vi "Teleop.vi"(10 "Match Info":T2={"Autonomous Elapsed Seconds"=0.0, "TeleOp Elapsed Seconds"=0.0, "Disabled Elapsed Seconds"=0.0, "Visited Autonomous"=FALSE, "Visited TeleOp"=FALSE, "Visited Disabled"=FALSE, "Autonomous Settings"={"Autonomous Style"=enum."Independent", "VI Refnum"=refnum}}, 11 "Call Context":T3) -> ()   [LabVIEW 2012]
doc: "This VI is called for each TeleOp packet received from the DS where the robot is not disabled. It is often used to read from the joysticks and update I/O or to update setpoints for timed control loops. It should complete and return within 20 milliseconds or it may miss DS packets."
uses:
  <vilib>/Rock Robotics/WPI/DriverStation/WPI_DriverStationDerivedRobotMode.ctl
  <vilib>/Rock Robotics/WPI/DriverStation/WPI_DriverStationMatch Info.ctl
  <vilib>/Rock Robotics/WPI/Relay/WPI_RelayValue.ctl
  <vilib>/Rock Robotics/WPI/Solenoid/WPI_SolenoidValue.ctl
  Robot Global Data.vi
  <vilib>/addons/control/pid/pid.llb/PID (DBL).vi
  <vilib>/Rock Robotics/WPI/RobotDrive/WPI_RobotDriveGetSetRefNum.vi
  <vilib>/Rock Robotics/WPI/Joystick/WPI_JoystickGetSetRefNum.vi
  <vilib>/Rock Robotics/WPI/Solenoid/WPI_SolenoidSetEnum.vi
  <vilib>/addons/control/pid/NI_PID_pid.lvlib
panel:
  in  "y 2":dbl=0.59
  in  "y":dbl=0.6
  in  "Boolean":bool
  in  "Time to twitch":dbl=1300.0
  in  "Time of start twitch":dbl
  in  "Turn speed for twitch":dbl=0.7
  in  "Twitch":string="Nope"
  in  "PID Gains Angle":T1={"proportional gain (Kc)"=1.0, "integral time (Ti, min)"=0.01, "derivative time (Td, min)"=0.0} {"derivative time (Td, min)" format="%.3f"; "integral time (Ti, min)" format="%.3f"; "proportional gain (Kc)" format="%.3f"}
  in  "PID Gains for distance":T1={"proportional gain (Kc)"=1.0, "integral time (Ti, min)"=0.01, "derivative time (Td, min)"=0.0} {"derivative time (Td, min)" format="%.3f"; "integral time (Ti, min)" format="%.3f"; "proportional gain (Kc)" format="%.3f"}
  in  "Threshold for shooter":dbl=0.015
  in  "Posistioned":string="Nothing"
  in  "Angle Target":dbl
  out "Distance From Target":dbl
  out "Ready To Fire":bool
  in  "S Off Time":dbl=0.5
  in  "S On Time":dbl=0.2
  in  "Time Last Fired":dbl
  in  "Current Status":string="Roaming"
  in  "Shooter Speed":dbl format="%.2f"
  in  "Shooter On":bool=TRUE
  out "Waveform Chart":cluster{"Rate":dbl, "Rate":dbl}(graph)
  out "Rate 1":dbl
  out "Rate 2":dbl
  in  "PID gains":T1={"proportional gain (Kc)"=1.0, "integral time (Ti, min)"=0.007, "derivative time (Td, min)"=0.0} {"derivative time (Td, min)" format="%.3f"; "integral time (Ti, min)" format="%.3f"; "proportional gain (Kc)" format="%.3f"}
  in  "Maximum Encoder speed":dbl=25000.0
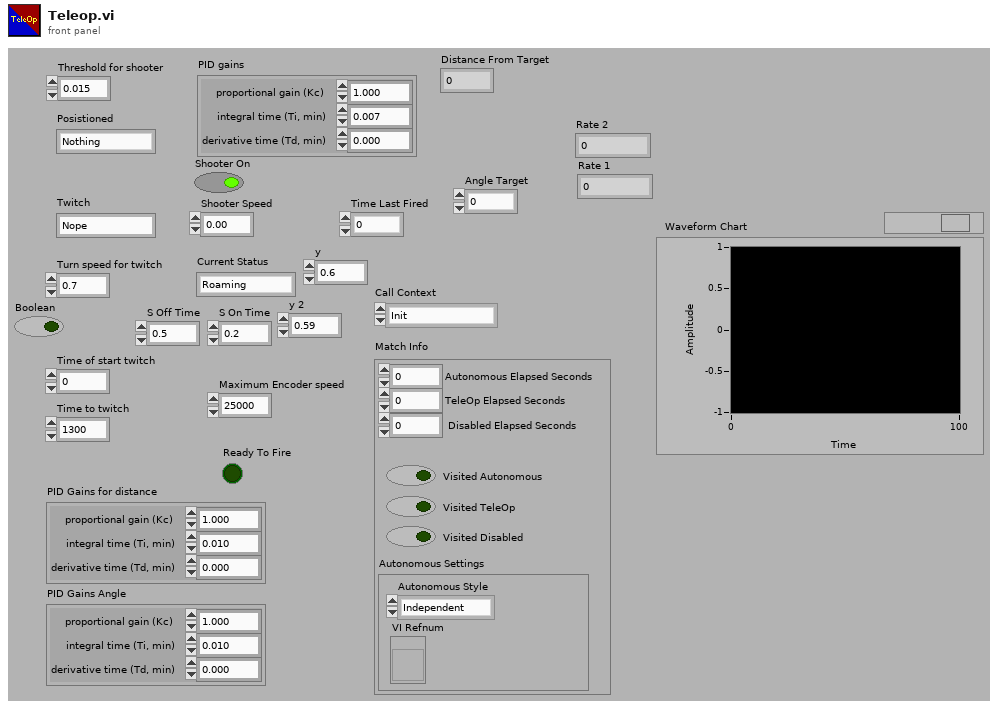
[diagram p1: front panel]
types:
  T1 = cluster{"proportional gain (Kc)":dbl, "integral time (Ti, min)":dbl, "derivative time (Td, min)":dbl}
  T2 = typedef "WPI_DriverStationMatch Info.ctl" = cluster{"Autonomous Elapsed Seconds":dbl, "TeleOp Elapsed Seconds":dbl, "Disabled Elapsed Seconds":dbl, "Visited Autonomous":bool, "Visited TeleOp":bool, "Visited Disabled":bool, "Autonomous Settings":cluster{"Autonomous Style":enum16{"Iterative", "Independent"}, "VI Refnum":refnum<vi>}}
  T3 = typedef "WPI_DriverStationDerivedRobotMode.ctl" = enum16{"Init", "Execute", "Stop"}
  T4 = typedef "WPI_EncoderDevRef.ctl" = cluster{"DevStatus":errorcluster, "EncoderIndex":T5, "CounterIndex":T6, "DistancePerCount":dbl, "Decoding Type":T7}
  T5 = typedef "FPGA_EncoderIdx.ctl" = enum8{"Enc 0", "Enc 1", "Enc 2", "Enc 3", "Invalid"}
  T6 = typedef "FPGA_CounterCtrSystemIndex.ctl" = enum8{"Ctr 0", "Ctr 1", "Ctr 2", "Ctr 3", "Ctr 4", "Ctr 5", "Ctr 6", "Ctr 7", "Invalid"}
  T7 = typedef "WPI_EncoderType.ctl" = enum16{"1x", "2x", "4x"}
  T8 = typedef "WPI_JoystickDevRef.ctl" = cluster{"Device":T9}
  T9 = typedef "WPI_JoystickDeviceEnum.ctl" = enum16{"USB 1", "USB 2", "USB 3", "USB 4", "Kinect 1", "Kinect 2"}
  T10 = typedef "WPI_JoystickButtonState.ctl" = cluster{"Button 1":bool, "Button 2":bool, "Button 3":bool, "Button 4":bool, "Button 5":bool, "Button 6":bool, "Button 7":bool, "Button 8":bool, "Button 9":bool, "Button 10":bool, "Button 11":bool, "Button 12":bool}
  T11 = typedef "WPI_RobotDriveDevRef.ctl" = cluster{"DevStatus":errorcluster, "Motors[]":T12[], "Square Inputs":bool, "Max Output":dbl, "Isochronous":bool}
  T12 = typedef "WPI_MotorControlDeviceRef.ctl" = cluster{"DeviceStatus":errorcluster, "Type":enum16{"PWM", "CAN"}, "PWM":cluster{"Digital Module":T13, "PWM Channel":T14, "DeadBand":T15}, "CAN":cluster{"Device Number":u8, "Control Mode":T16, "Semaphore":T17, "Max Vout":dbl}, "Invert":bool, "TransformRef":T18, "InvTransformRef":T18}
  T13 = typedef "FPGA_TypedefDigitalModule.ctl" = enum16{"Digital Module 1", "Digital Module 2"}
  T14 = typedef "FPGA_DIOPWMChannel.ctl" = enum8{"PWM 1", "PWM 2", "PWM 3", "PWM 4", "PWM 5", "PWM 6", "PWM 7", "PWM 8", "PWM 9", "PWM 10", "Invalid"}
  T15 = typedef "WPI_PWMDeadband.ctl" = cluster{"Name":string, "maxPositivePwm":i32, "minPositivePwm":i32, "centerPwm":i32, "maxNegativePwm":i32, "minNegativePwm":i32, "angularRange":u16}
  T16 = typedef "WPI_CANJaguar_ControlMode.ctl" = enum8{"Percent VBus", "Current", "Speed", "Position", "Voltage"}
  T17 = typedef "Semaphore RefNum" = refnum<k1>
  T18 = typedef "WPI_PWMTransform_ConPane.ctl" = refnum<vi>
  T19 = cluster{"axis 1 (x)":dbl, "axis 2 (y)":dbl, "axis 3 (throttle)":dbl, "axis 4":dbl, "axis 5":dbl, "axis 6":dbl}
  T20 = typedef "WPI_RelayValue.ctl" = enum16{"Off", "On", "Forward", "Reverse"}
  T21 = typedef "WPI_RelayDevRef.ctl" = cluster{"DevStatus":errorcluster, "Relay Channel":T22, "Digital Module":T13, "Relay Direction":T23}
  T22 = typedef "FPGA_DIORelayChannel.ctl" = enum8{"Relay 1", "Relay 2", "Relay 3", "Relay 4", "Relay 5", "Relay 6", "Relay 7", "Relay 8", "Invalid"}
  T23 = typedef "WPI_RelayDirection.ctl" = enum16{"Both directions", "Forward only", "Reverse only"}
  T24 = typedef "WPI_SolenoidValue.ctl" = enum16{"Off", "On", "Forward", "Reverse"}
  T25 = typedef "WPI_SolenoidDevRef.ctl" = cluster{"DevStatus":errorcluster, "Solenoid Module":T26, "Forward Solenoid Channel":T27, "Reverse Solenoid Channel":T27}
  T26 = typedef "FPGA_TypedefSolenoidModule.ctl" = enum16{"Solenoid Module 1", "Solenoid Module 2"}
  T27 = typedef "WPI_SolenoidChannel.ctl" = enum8{"Solenoid 1", "Solenoid 2", "Solenoid 3", "Solenoid 4", "Solenoid 5", "Solenoid 6", "Solenoid 7", "Solenoid 8", "Invalid"}
  T28 = cluster{"Center Position":cluster{"X":dbl, "Y":dbl}, "Distance (ft)":dbl, "Center":bool}[]
  T29 = cluster{"Center Position":cluster{"X":dbl, "Y":dbl}, "Distance (ft)":dbl, "Center":bool}
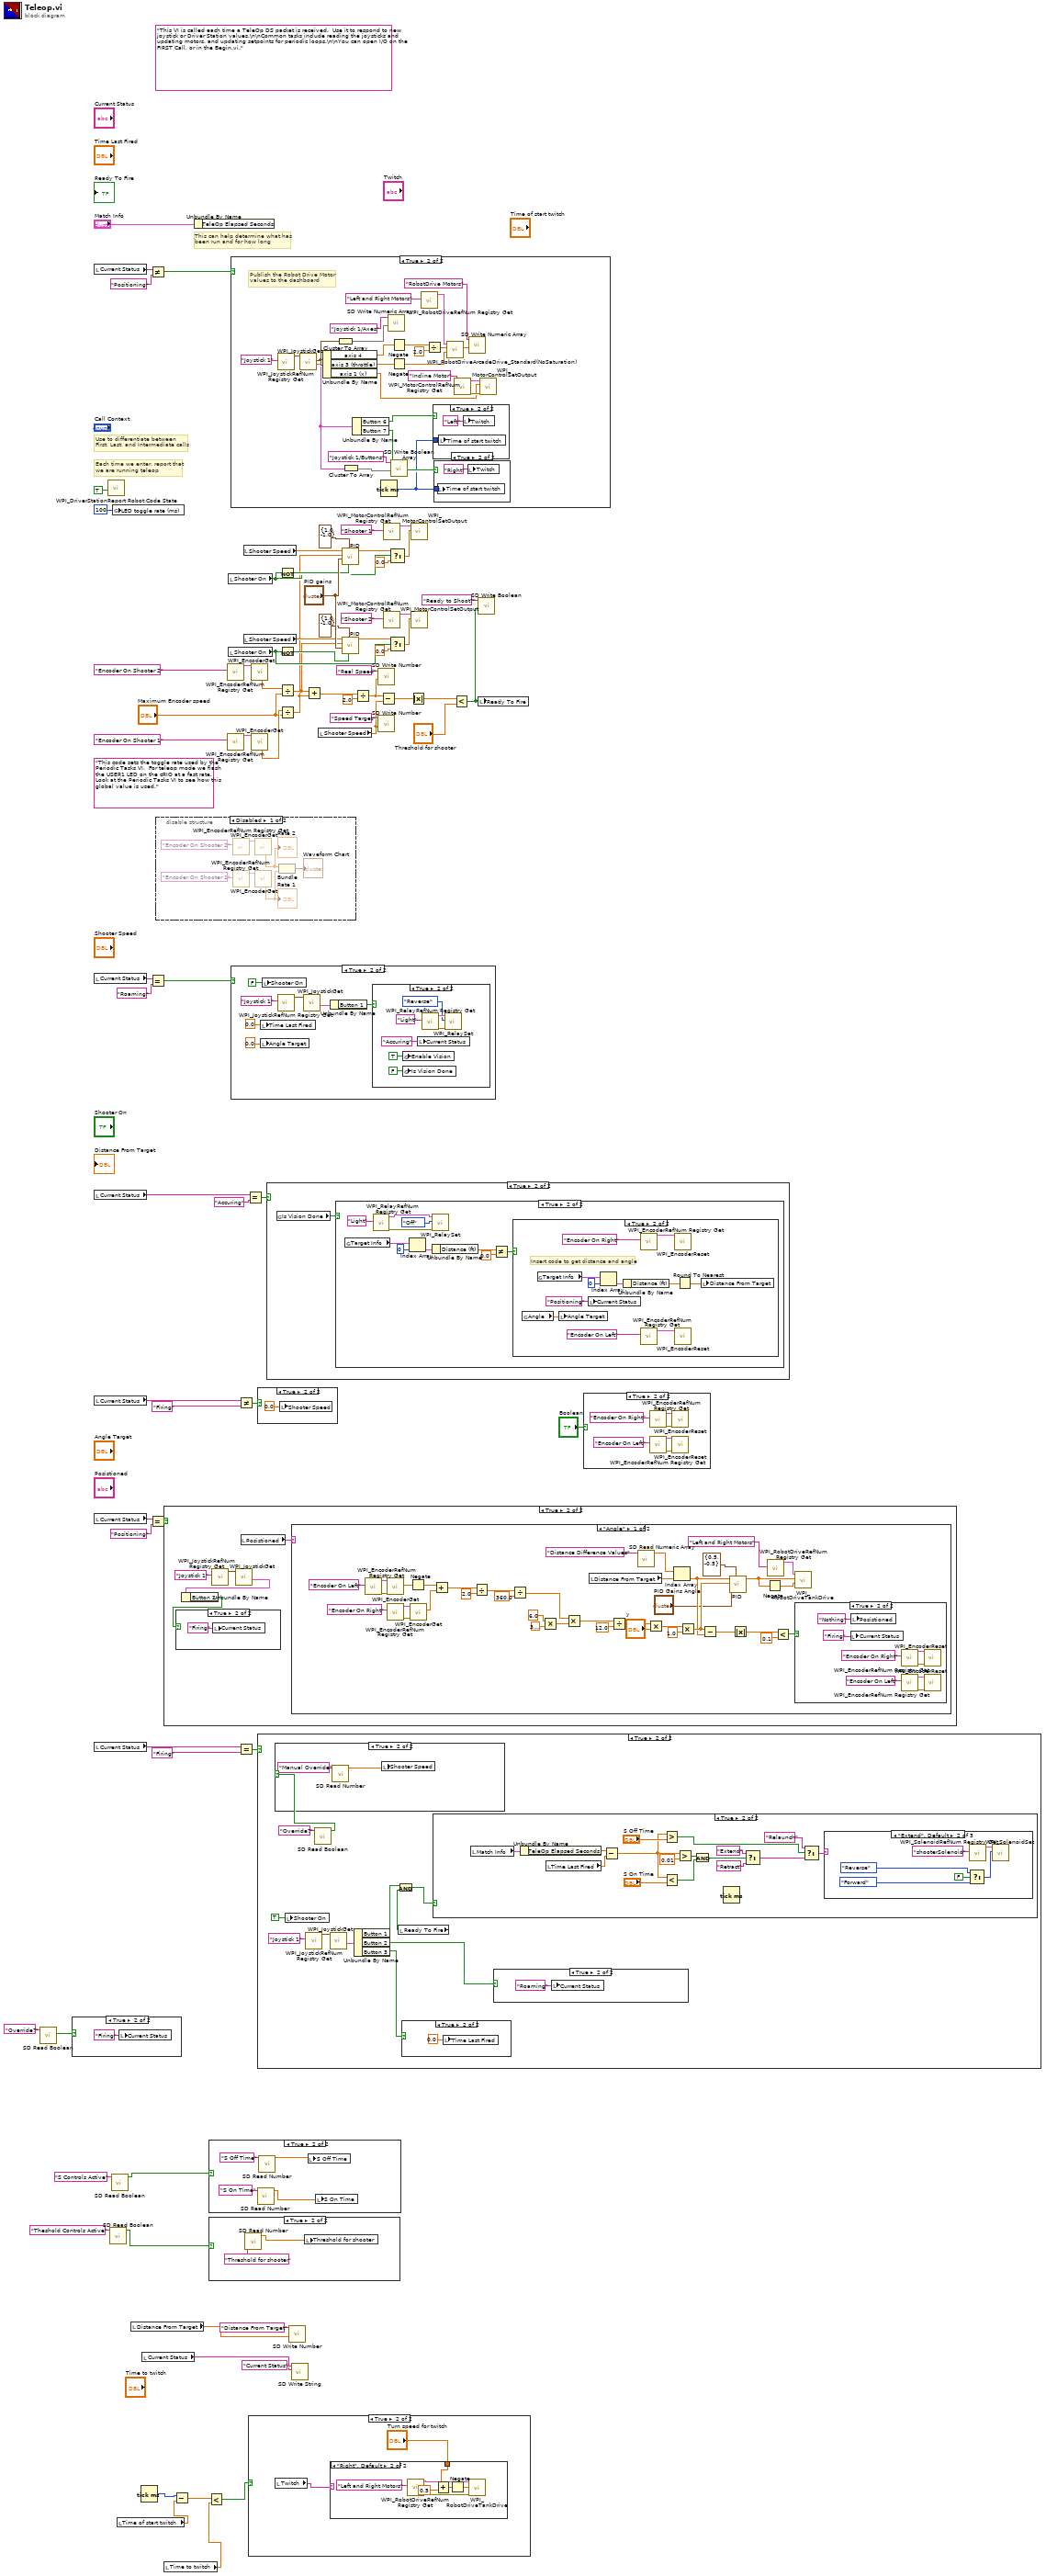
[diagram p0: block diagram]
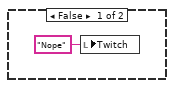
[diagram p3: hidden frame]
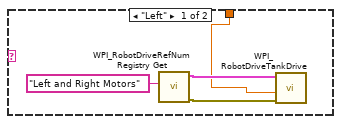
[diagram p4: hidden frame]
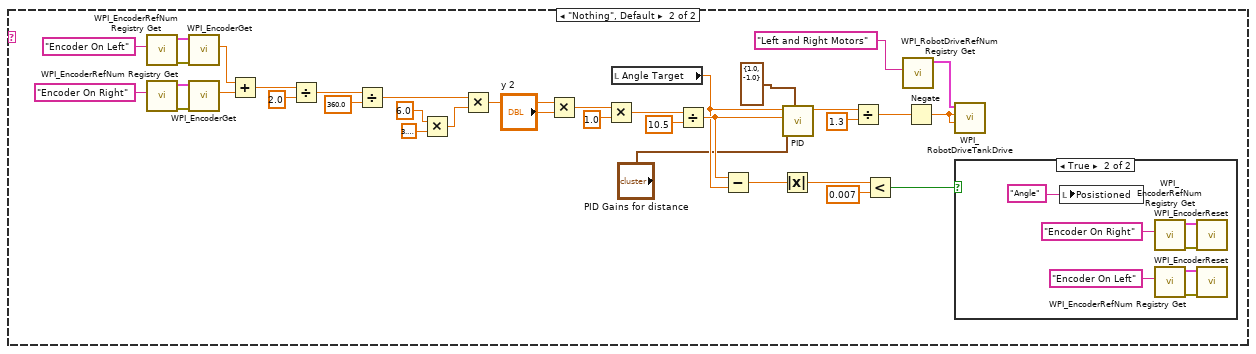
[diagram p12: hidden frame]
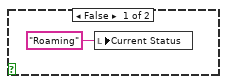
[diagram p19: hidden frame]
diagram:
  (unwired) "This code sets the toggle rate used by the Periodic Tasks VI.  For teleop mode we flash the USER1 LED on the cRIO at a fast rate.  Look at the Periodic Tasks VI to see how this global value is used."
  (unwired) "This VI is called each time a TeleOp DS packet is received.  Use it to respond to new joystick or Driver Station values.\n\nCommon tasks include reading the joysticks and updating motors, and updating setpoints for periodic loops.\n\nYou can open I/O on the FIRST Call, or in the Begin.vi."
  # "Each time we enter, report that\nwe are running teleop"
  # "Use to differentiate between\nFirst, Last, and Intermediate calls"
  # "This can help determine what has\nbeen run and for how long"
  n1 = call <vilib>:"SD Read Boolean.vi"("Name"="Override?") -> ("Boolean"=w15:bool)  [unwired: 8 in, 2 out]
  n2 = case shown="True" w15 {
    frame False {
    }
    frame True {
      n3 = local write "Current Status"("Firing" ("Current Status")) -> ()
    }
  }
  n4 = local read "Current Status"() -> (w26:string)
  n5 = local read "Current Status"() -> (w32:string)
  n6 = local read "Current Status"() -> (w29:string)
  n7 = local read "Current Status"() -> (w19:string)
  n8 = local read "Current Status"() -> (w23:string)
  n9 = local read "Current Status"() -> (w47:string)
  n10 = call <vilib>:"WPI_DriverStationReport Robot Code State.vi"("TeleOp"=TRUE ("Autonomous")) -> ()  [unwired: 10 in, 1 out]
  n11 = call <vilib>:"SD Read Boolean.vi"("Name"="Theshold Controls Active") -> ("Boolean"=w14:bool)  [unwired: 8 in, 2 out]
  n12 = call <vilib>:"SD Read Boolean.vi"("Name"="S Controls Active") -> ("Boolean"=w12:bool)  [unwired: 8 in, 2 out]
  n13 = global write "Robot Global Data.vi" "LED toggle rate (ms)"(u32 100 ("LED ms toggle rate")) -> ()
  n14 = local read "Time of start twitch"() -> (w5:dbl)
  n15 = local read "Distance From Target"() -> (w9:dbl)
  n16 = Tick Count (ms)() -> (millisecond timer value=w6:u32)
  n17 = local read "Current Status"() -> (w7:string)
  n18 = Not Equal?(x=w26, y="Positioning") -> (x != y?=w24:bool)
  n19 = Equal?(x=w32, y="Roaming") -> (x = y?=w30:bool)
  n20 = Equal?(x=w23, y="Positioning") -> (x = y?=w21:bool)
  n21 = disable-structure shown="Disabled" {
    frame Disabled {
      n22 = call <vilib>:"WPI_EncoderRefNum Registry Get.vi"("refnum name"="Encoder On Shooter 2") -> ("EncoderDevRef"=w83:T4)  [unwired: 9 in, 1 out]
      n23 = call <vilib>:"WPI_EncoderRefNum Registry Get.vi"("refnum name"="Encoder On Shooter 1") -> ("EncoderDevRef"=w82:T4)  [unwired: 9 in, 1 out]
      n24 = call <vilib>:"WPI_EncoderGet.vi"("EncoderDevRef"=w83) -> ("Rate"=w80:dbl)  [unwired: 5 in, 5 out]
      "Rate 2" <- w80
      n25 = call <vilib>:"WPI_EncoderGet.vi"("EncoderDevRef"=w82) -> ("Rate"=w81:dbl)  [unwired: 5 in, 5 out]
      "Rate 1" <- w81
      n26 = Bundle("Rate"=w80, "Rate"=w81) -> (→"Waveform Chart":cluster{"Rate":dbl, "Rate":dbl})  [unwired: 1 in]
    }
    frame Enabled {
    }
  }
  n27 = case shown="True" w21 {
    frame False {
    }
    frame True {
      n28 = call <vilib>:"WPI_JoystickRefNum Registry Get.vi"("refnum name"="Joystick 1") -> ("JoystickDevRef"=w87:T8)  [unwired: 9 in, 1 out]
      n29 = call <vilib>:"WPI_JoystickGet.vi"("JoystickDevRef"=w87) -> ("Buttons"=w86:T10)  [unwired: 4 in, 2 out]
      n30 = Unbundle By Name(w86) -> ("Button 2"=w85:bool)
      n31 = case shown="True" w85 {
        frame False {
        }
        frame True {
          n32 = local write "Current Status"("Firing" ("Current Status")) -> ()
        }
      }
      n33 = local read "Posistioned"() -> (w89:string)
      n34 = case shown="\"Angle\"" w89 {
        frame "Angle" {
          n35 = call <vilib>:"WPI_EncoderRefNum Registry Get.vi"("refnum name"="Encoder On Left") -> ("error out"=w104:errorcluster, "EncoderDevRef"=w105:T4)  [unwired: 9 in]
          n36 = call <vilib>:"WPI_EncoderGet.vi"("error in (no error)"=w104, "EncoderDevRef"=w105) -> ("Distance"=w97:dbl)  [unwired: 4 in, 5 out]
          n37 = call <vilib>:"WPI_EncoderRefNum Registry Get.vi"("refnum name"="Encoder On Right") -> ("error out"=w106:errorcluster, "EncoderDevRef"=w107:T4)  [unwired: 9 in]
          n38 = Negate(x=w97) -> (-x=w96:dbl)
          n39 = call <vilib>:"WPI_EncoderGet.vi"("error in (no error)"=w106, "EncoderDevRef"=w107) -> ("Distance"=w110:dbl)  [unwired: 4 in, 5 out]
          n40 = Add(x=w96, y=w110) -> (x+y=w111:dbl)
          n41 = Divide(x=w111, y=2.0) -> (x/y=w115:dbl)
          n42 = Divide(x=w115, y=360.0) -> (x/y=w117:dbl)
          n43 = Multiply(x=6.0, y=3.141592653589793) -> (x*y=w118:dbl)
          n44 = Multiply(x=w117, y=w118) -> (x*y=w119:dbl)
          n45 = local read "Distance From Target"() -> (w94:dbl)
          n46 = Divide(x=w119, y=12.0) -> (x/y=w100:dbl)
          n47 = call <vilib>:"SD Read Numeric Array.vi"("Name"="Distance Difference Values") -> ("Numeric Array"=w124:dbl[])  [unwired: 8 in, 2 out]
          n48 = Multiply(x=w100, y="y") -> (x*y=w99:dbl)
          n49 = Index Array(array=w124, index=w94) -> (element=w93:dbl)
          n50 = Multiply(x=w99, y=1.0) -> (x*y=w95:dbl)
          n51 = Subtract(x=w95, y=w93) -> (x-y=w125:dbl)
          n52 = call-poly <vilib>:"PID.vi"("output range"=cluster{"output high":dbl, "output low":dbl} {"output high"=0.5, "output low"=-0.5}, "PID gains"="PID Gains Angle", "process variable"=w95, "setpoint"=w93) -> ("output"=w101:dbl)  [unwired: 6 in, 1 out]
          n53 = Absolute Value(x=w125) -> (abs(x)=w126:dbl)
          n54 = Negate(x=w101) -> (-x=w103:dbl)
          n55 = call <vilib>:"WPI_RobotDriveRefNum Registry Get.vi"("refnum name"="Left and Right Motors") -> ("RobotDriveDevRef"=w122:T11)  [unwired: 9 in, 1 out]
          n56 = Less?(x=w126, y=0.1) -> (x < y?=w128:bool)
          n57 = call <vilib>:"WPI_RobotDriveTankDrive.vi"("Right axis value"=w103, "Left axis value"=w101, "RobotDriveDevRef"=w122) -> ()  [unwired: 6 in, 3 out]
          n58 = case shown="True" w128 {
            frame False {
            }
            frame True {
              n59 = local write "Current Status"("Firing" ("Current Status")) -> ()
              n60 = local write "Posistioned"("Nothing" ("Posistioned")) -> ()
              n61 = call <vilib>:"WPI_EncoderRefNum Registry Get.vi"("refnum name"="Encoder On Right") -> ("error out"=w134:errorcluster, "EncoderDevRef"=w135:T4)  [unwired: 9 in]
              n62 = call <vilib>:"WPI_EncoderRefNum Registry Get.vi"("refnum name"="Encoder On Left") -> ("error out"=w132:errorcluster, "EncoderDevRef"=w133:T4)  [unwired: 9 in]
              n63 = call <vilib>:"WPI_EncoderReset.vi"("error in (no error)"=w134, "EncoderDevRef"=w135) -> ()  [unwired: 8 in, 2 out]
              n64 = call <vilib>:"WPI_EncoderReset.vi"("error in (no error)"=w132, "EncoderDevRef"=w133) -> ()  [unwired: 8 in, 2 out]
            }
          }
        }
        frame "Nothing", Default {
          n65 = call <vilib>:"WPI_EncoderRefNum Registry Get.vi"("refnum name"="Encoder On Left") -> ("error out"=w172:errorcluster, "EncoderDevRef"=w171:T4)  [unwired: 9 in]
          n66 = call <vilib>:"WPI_EncoderRefNum Registry Get.vi"("refnum name"="Encoder On Right") -> ("error out"=w170:errorcluster, "EncoderDevRef"=w169:T4)  [unwired: 9 in]
          n67 = call <vilib>:"WPI_EncoderGet.vi"("error in (no error)"=w172, "EncoderDevRef"=w171) -> ("Distance"=w166:dbl)  [unwired: 4 in, 5 out]
          n68 = call <vilib>:"WPI_EncoderGet.vi"("error in (no error)"=w170, "EncoderDevRef"=w169) -> ("Distance"=w148:dbl)  [unwired: 4 in, 5 out]
          n69 = Add(x=w166, y=w148) -> (x+y=w165:dbl)
          n70 = Divide(x=w165, y=2.0) -> (x/y=w161:dbl)
          n71 = Divide(x=w161, y=360.0) -> (x/y=w154:dbl)
          n72 = Multiply(x=6.0, y=3.141592653589793) -> (x*y=w159:dbl)
          n73 = Multiply(x=w154, y=w159) -> (x*y=w143:dbl)
          n74 = Multiply(x=w143, y="y 2") -> (x*y=w142:dbl)
          n75 = Multiply(x=w142, y=1.0) -> (x*y=w141:dbl)
          n76 = local read "Angle Target"() -> (w139:dbl)
          n77 = Divide(x=w141, y=10.5) -> (x/y=w150:dbl)
          n78 = Subtract(x=w150, y=w139) -> (x-y=w151:dbl)
          n79 = Absolute Value(x=w151) -> (abs(x)=w152:dbl)
          n80 = call-poly <vilib>:"PID.vi"("output range"=cluster{"output high":dbl, "output low":dbl} {"output high"=1.0, "output low"=-1.0}, "PID gains"="PID Gains for distance", "process variable"=w150, "setpoint"=w139) -> ("output"=w155:dbl)  [unwired: 6 in, 1 out]
          n81 = Divide(x=w155, y=1.3) -> (x/y=w147:dbl)
          n82 = Less?(x=w152, y=0.007) -> (x < y?=w145:bool)
          n83 = call <vilib>:"WPI_RobotDriveRefNum Registry Get.vi"("refnum name"="Left and Right Motors") -> ("RobotDriveDevRef"=w156:T11)  [unwired: 9 in, 1 out]
          n84 = Negate(x=w147) -> (-x=w146:dbl)
          n85 = call <vilib>:"WPI_RobotDriveTankDrive.vi"("Right axis value"=w146, "Left axis value"=w146, "RobotDriveDevRef"=w156) -> ()  [unwired: 6 in, 3 out]
          n86 = case shown="True" w145 {
            frame False {
            }
            frame True {
              n87 = local write "Posistioned"("Angle" ("Posistioned")) -> ()
              n88 = call <vilib>:"WPI_EncoderRefNum Registry Get.vi"("refnum name"="Encoder On Right") -> ("error out"=w175:errorcluster, "EncoderDevRef"=w174:T4)  [unwired: 9 in]
              n89 = call <vilib>:"WPI_EncoderRefNum Registry Get.vi"("refnum name"="Encoder On Left") -> ("error out"=w177:errorcluster, "EncoderDevRef"=w176:T4)  [unwired: 9 in]
              n90 = call <vilib>:"WPI_EncoderReset.vi"("error in (no error)"=w175, "EncoderDevRef"=w174) -> ()  [unwired: 8 in, 2 out]
              n91 = call <vilib>:"WPI_EncoderReset.vi"("error in (no error)"=w177, "EncoderDevRef"=w176) -> ()  [unwired: 8 in, 2 out]
            }
          }
        }
      }
    }
  }
  n92 = local read "Time to twitch"() -> (w3:dbl)
  n93 = Subtract(x=w6, y=w5) -> (x-y=w4:dbl)
  n94 = Unbundle By Name("Match Info") -> ()  [unwired: 1 out]
  n95 = Less?(x=w4, y=w3) -> (x < y?=w2:bool)
  n96 = case shown="True" w12 {
    frame False {
    }
    frame True {
      n97 = call <vilib>:"SD Read Number.vi"("Name"="S On Time") -> ("Numeric"=w182:dbl)  [unwired: 8 in, 2 out]
      n98 = call <vilib>:"SD Read Number.vi"("Name"="S Off Time") -> ("Numeric"=w183:dbl)  [unwired: 8 in, 2 out]
      n99 = local write "S Off Time"(w183) -> ()
      n100 = local write "S On Time"(w182) -> ()
    }
  }
  n101 = case shown="True" w14 {
    frame False {
    }
    frame True {
      n102 = call <vilib>:"SD Read Number.vi"("Name"="Threshold for shooter") -> ("Numeric"=w184:dbl)  [unwired: 8 in, 2 out]
      n103 = local write "Threshold for shooter"(w184) -> ()
    }
  }
  n104 = call <vilib>:"WPI_EncoderRefNum Registry Get.vi"("refnum name"="Encoder On Shooter 2") -> ("EncoderDevRef"=w61:T4)  [unwired: 9 in, 1 out]
  n105 = call <vilib>:"WPI_EncoderRefNum Registry Get.vi"("refnum name"="Encoder On Shooter 1") -> ("EncoderDevRef"=w70:T4)  [unwired: 9 in, 1 out]
  n106 = local read "Shooter On"() -> (w50:bool)
  n107 = local read "Shooter On"() -> (w51:bool)
  n108 = case shown="True" w24 {
    frame False {
    }
    frame True {
      # "Publish the Robot Drive Motor\nvalues to the dashboard"
      n109 = call <vilib>:"WPI_JoystickRefNum Registry Get.vi"("refnum name"="Joystick 1") -> ("JoystickDevRef"=w203:T8)  [unwired: 1 in, 9 out]
      n110 = call <vilib>:"WPI_JoystickGet.vi"("JoystickDevRef"=w203) -> ("Buttons"=w189:T10, "Axes"=w206:T19)  [unwired: 1 in, 4 out]
      n111 = Unbundle By Name(w206) -> ("axis 4"=w199:dbl, "axis 3 (throttle)"=w197:dbl, "axis 1 (x)"=w190:dbl)
      n112 = Cluster To Array(cluster=w206) -> (array=w207:dbl[])
      n113 = Cluster To Array(cluster=w189) -> (array=w204:bool[])
      n114 = Unbundle By Name(w189) -> ("Button 6"=w188:bool, "Button 7"=w187:bool)
      n115 = Tick Count (ms)() -> (millisecond timer value=w186:u32)
      n116 = call <vilib>:"SD Write Numeric Array.vi"("Numeric Array"=w207, "Name"="Joystick 1/Axes") -> ()  [unwired: 8 in, 2 out]
      n117 = Negate(x=w199) -> (-x=w196:dbl)
      n118 = Negate(x=w197) -> (-x=w198:dbl)
      n119 = call <vilib>:"SD Write Boolean Array.vi"("Boolean Array"=w204, "Name"="Joystick 1/Buttons") -> ()  [unwired: 8 in, 2 out]
      n120 = call <vilib>:"WPI_RobotDriveRefNum Registry Get.vi"("refnum name"="Left and Right Motors") -> ("RobotDriveDevRef"=w202:T11)  [unwired: 1 in, 9 out]
      n121 = Divide(x=w196, y=2.0) -> (x/y=w194:dbl)
      n122 = case shown="True" w188 {
        tunnel: w186 -> [_ w211]
        frame False {
        }
        frame True {
          n123 = local write "Time of start twitch"(w211) -> ()
          n124 = local write "Twitch"("Left" ("Twitch")) -> ()
        }
      }
      n125 = case shown="True" w187 {
        tunnel: w186 -> [_ w213]
        frame False {
        }
        frame True {
          n126 = local write "Time of start twitch"(w213) -> ()
          n127 = local write "Twitch"("Right" ("Twitch")) -> ()
        }
      }
      n128 = call <vilib>:"WPI_RobotDriveArcadeDrive_Standard(NoSaturation).vi"("Y axis value"=w198, "X axis value"=w194, "RobotDriveDevRef"=w202) -> ("Motor Values"=w210:dbl[])  [unwired: 1 in, 7 out]
      n129 = call <vilib>:"WPI_MotorControlRefNum Registry Get.vi"("refnum name"="Incline Motor") -> ("error out"=w192:errorcluster, "MotorControlDevRef"=w191:T12)  [unwired: 9 in]
      n130 = call <vilib>:"SD Write Numeric Array.vi"("Numeric Array"=w210, "Name"="RobotDrive Motors") -> ()  [unwired: 8 in, 2 out]
      n131 = call <vilib>:"WPI_MotorControlSetOutput.vi"("error in (no error)"=w192, "Output"=w190, "MotorControlDevRef"=w191) -> ()  [unwired: 6 in, 3 out]
    }
  }
  n132 = case shown="True" w30 {
    frame False {
    }
    frame True {
      n133 = local write "Time Last Fired"(0.0 ("Time Last Fired")) -> ()
      n134 = local write "Angle Target"(0.0 ("Angle Target")) -> ()
      n135 = local write "Shooter On"(FALSE ("Shooter On")) -> ()
      n136 = call <vilib>:"WPI_JoystickRefNum Registry Get.vi"("refnum name"="Joystick 1") -> ("JoystickDevRef"=w220:T8)  [unwired: 9 in, 1 out]
      n137 = call <vilib>:"WPI_JoystickGet.vi"("JoystickDevRef"=w220) -> ("Buttons"=w219:T10)  [unwired: 4 in, 2 out]
      n138 = Unbundle By Name(w219) -> ("Button 1"=w218:bool)
      n139 = case shown="True" w218 {
        frame False {
        }
        frame True {
          n140 = global write "Robot Global Data.vi" "Enable Vision"(TRUE ("Enable Vision")) -> ()
          n141 = global write "Robot Global Data.vi" "Is Vision Done"(FALSE ("Is Vision Done")) -> ()
          n142 = local write "Current Status"("Accuring" ("Current Status")) -> ()
          n143 = call <vilib>:"WPI_RelayRefNum Registry Get.vi"("refnum name"="Light") -> ("error out"=w224:errorcluster, "RelayDevRef"=w225:T21)  [unwired: 9 in]
          n144 = call <vilib>:"WPI_RelaySet.vi"("error in (no error)"=w224, "RelayValue"=WPI_RelayValue."Reverse", "RelayDevRef"=w225) -> ()  [unwired: 7 in, 2 out]
        }
      }
    }
  }
  n145 = Not Equal?(x=w19, y="Firing") -> (x != y?=w18:bool)
  n146 = Equal?(x=w47, y="Firing") -> (x = y?=w45:bool)
  n147 = local read "Shooter Speed"() -> (w49:dbl)
  n148 = local read "Shooter Speed"() -> (w48:dbl)
  n149 = Equal?(x=w29, y="Accuring") -> (x = y?=w27:bool)
  n150 = case shown="True" w2 {
    frame False {
      n151 = local write "Twitch"("Nope" ("Twitch")) -> ()
    }
    frame True {
      n152 = local read "Twitch"() -> (w230:string)
      n153 = case shown="\"Right\", Default" w230 {
        tunnel: "Turn speed for twitch" -> [w232 w238]
        frame "Left" {
          n154 = call <vilib>:"WPI_RobotDriveRefNum Registry Get.vi"("refnum name"="Left and Right Motors") -> ("error out"=w235:errorcluster, "RobotDriveDevRef"=w234:T11)  [unwired: 9 in]
          n155 = call <vilib>:"WPI_RobotDriveTankDrive.vi"("error in (no error)"=w235, "Right axis value"=w232, "RobotDriveDevRef"=w234) -> ()  [unwired: 6 in, 3 out]
        }
        frame "Right", Default {
          n156 = call <vilib>:"WPI_RobotDriveRefNum Registry Get.vi"("refnum name"="Left and Right Motors") -> ("error out"=w242:errorcluster, "RobotDriveDevRef"=w241:T11)  [unwired: 9 in]
          n157 = Add(x=w238, y=0.5) -> (x+y=w236:dbl)
          n158 = Negate(x=w236) -> (-x=w239:dbl)
          n159 = call <vilib>:"WPI_RobotDriveTankDrive.vi"("error in (no error)"=w242, "Left axis value"=w239, "RobotDriveDevRef"=w241) -> ()  [unwired: 6 in, 3 out]
        }
      }
    }
  }
  n160 = call <vilib>:"WPI_EncoderGet.vi"("EncoderDevRef"=w61) -> ("Rate"=w53:dbl)  [unwired: 5 in, 5 out]
  n161 = call <vilib>:"WPI_EncoderGet.vi"("EncoderDevRef"=w70) -> ("Rate"=w54:dbl)  [unwired: 5 in, 5 out]
  n162 = case shown="True" w18 {
    frame False {
    }
    frame True {
      n163 = local write "Shooter Speed"(0.0 ("Shooter Speed")) -> ()
    }
  }
  n164 = case shown="True" w45 {
    frame False {
    }
    frame True {
      n165 = local write "Shooter On"(TRUE ("Shooter On")) -> ()
      n166 = call <vilib>:"WPI_JoystickRefNum Registry Get.vi"("refnum name"="Joystick 1") -> ("JoystickDevRef"=w253:T8)  [unwired: 9 in, 1 out]
      n167 = call <vilib>:"SD Read Boolean.vi"("Name"="Override?") -> ("Boolean"=w244:bool)  [unwired: 8 in, 2 out]
      n168 = case shown="True" w244 {
        frame False {
          n169 = local read "Distance From Target"() -> (w255:dbl)
          n170 = call <vilib>:"SD Read Numeric Array.vi"("Name"="Speed Values") -> ("Numeric Array"=w257:dbl[])  [unwired: 8 in, 2 out]
          n171 = Index Array(array=w257, index=w255) -> (element=w256:dbl)
          n172 = local write "Shooter Speed"(w256) -> ()
        }
        frame True {
          n173 = call <vilib>:"SD Read Number.vi"("Name"="Manual Override") -> ("Numeric"=w259:dbl)  [unwired: 8 in, 2 out]
          n174 = local write "Shooter Speed"(w259) -> ()
        }
      }
      n175 = call <vilib>:"WPI_JoystickGet.vi"("JoystickDevRef"=w253) -> ("Buttons"=w252:T10)  [unwired: 4 in, 2 out]
      n176 = Unbundle By Name(w252) -> ("Button 1"=w251:bool, "Button 2"=w247:bool, "Button 3"=w246:bool)
      n177 = local read "Ready To Fire"() -> (w249:bool)
      n178 = And(x=w251, y=w249) -> (x .and. y?=w250:bool)
      n179 = case shown="True" w246 {
        frame False {
        }
        frame True {
          n180 = local write "Time Last Fired"(0.0 ("Time Last Fired")) -> ()
        }
      }
      n181 = case shown="True" w250 {
        frame False {
        }
        frame True {
          n182 = local read "Match Info"() -> (w278:T2)
          n183 = Unbundle By Name(w278) -> ("TeleOp Elapsed Seconds"=w277:dbl)
          n184 = local read "Time Last Fired"() -> (w276:dbl)
          n185 = Subtract(x=w277, y=w276) -> (x-y=w269:dbl)
          n186 = Greater?(x=w269, y="S Off Time") -> (0:w272:bool)
          n187 = Less?(x=w269, y="S On Time") -> (x < y?=w266:bool)
          n188 = Greater?(x=w269, y=0.01) -> (0:w267:bool)
          n189 = And(x=w267, y=w266) -> (x .and. y?=w265:bool)
          n190 = Tick Count (ms)() -> ()  [unwired: 1 out]
          n191 = Select(t="Extend" ("f"), s=w265, f="Retract") -> (s? t:f=w270:string)
          n192 = Select(t="Relaunch" ("f"), s=w272, f=w270) -> (s? t:f=w274:string)
          n193 = case shown="\"Extend\", Default" w274 {
            frame "Retract" {
              n194 = Select(t=WPI_SolenoidValue."Reverse" ("Value"), s=TRUE, f=WPI_SolenoidValue."Forward" ("Value")) -> (s? t:f=w283:T24)
              n195 = call <vilib>:"WPI_SolenoidRefNum Registry Get.vi"("refnum name"="shooterSolenoid") -> ("SolenoidDevRef"=w279:T25)  [unwired: 9 in, 1 out]
              n196 = call-poly <vilib>:"WPI_SolenoidSet.vi"("Value"=w283, "SolenoidDevRef"=w279) -> ()  [unwired: 8 in, 2 out]
            }
            frame "Extend", Default {
              n197 = Select(t=WPI_SolenoidValue."Reverse" ("Value"), s=FALSE, f=WPI_SolenoidValue."Forward" ("Value")) -> (s? t:f=w289:T24)
              n198 = call <vilib>:"WPI_SolenoidRefNum Registry Get.vi"("refnum name"="shooterSolenoid") -> ("SolenoidDevRef"=w285:T25)  [unwired: 9 in, 1 out]
              n199 = call-poly <vilib>:"WPI_SolenoidSet.vi"("Value"=w289, "SolenoidDevRef"=w285) -> ()  [unwired: 8 in, 2 out]
            }
            frame "Relaunch" {
              n200 = local read "Match Info"() -> (w292:T2)
              n201 = Unbundle By Name(w292) -> ("TeleOp Elapsed Seconds"=w291:dbl)
              n202 = local write "Time Last Fired"(w291) -> ()
            }
          }
        }
      }
      n203 = case shown="True" w247 {
        frame False {
        }
        frame True {
          n204 = local write "Current Status"("Roaming" ("Current Status")) -> ()
        }
      }
    }
  }
  n205 = case shown="True" w27 {
    frame False {
    }
    frame True {
      n206 = global read "Robot Global Data.vi" "Is Vision Done"() -> (w293:bool)
      n207 = case shown="True" w293 {
        frame False {
        }
        frame True {
          n208 = global read "Robot Global Data.vi" "Target Info"() -> (w303:T28)
          n209 = call <vilib>:"WPI_RelayRefNum Registry Get.vi"("refnum name"="Light") -> ("error out"=w296:errorcluster, "RelayDevRef"=w297:T21)  [unwired: 9 in]
          n210 = Index Array(array=w303, index=0) -> (element=w301:T29)
          n211 = call <vilib>:"WPI_RelaySet.vi"("error in (no error)"=w296, "RelayValue"=WPI_RelayValue."Off", "RelayDevRef"=w297) -> ()  [unwired: 7 in, 2 out]
          n212 = Unbundle By Name(w301) -> ("Distance (ft)"=w299:dbl)
          n213 = Not Equal?(x=w299, y=0.0) -> (x != y?=w300:bool)
          n214 = case shown="True" w300 {
            frame False {
              n215 = local write "Current Status"("Roaming" ("Current Status")) -> ()
            }
            frame True {
              # "Insert code to get distance and angle"
              n216 = global read "Robot Global Data.vi" "Angle"() -> (w310:dbl)
              n217 = global read "Robot Global Data.vi" "Target Info"() -> (w309:T28)
              n218 = local write "Angle Target"(w310) -> ()
              n219 = local write "Current Status"("Positioning" ("Current Status")) -> ()
              n220 = Index Array(array=w309, index=0) -> (element=w307:T29)
              n221 = Unbundle By Name(w307) -> ("Distance (ft)"=w306:dbl)
              n222 = call <vilib>:"WPI_EncoderRefNum Registry Get.vi"("refnum name"="Encoder On Right") -> ("EncoderDevRef"=w312:T4)  [unwired: 9 in, 1 out]
              n223 = call <vilib>:"WPI_EncoderRefNum Registry Get.vi"("refnum name"="Encoder On Left") -> ("EncoderDevRef"=w313:T4)  [unwired: 9 in, 1 out]
              n224 = call <vilib>:"WPI_EncoderReset.vi"("EncoderDevRef"=w312) -> ()  [unwired: 9 in, 2 out]
              n225 = call <vilib>:"WPI_EncoderReset.vi"("EncoderDevRef"=w313) -> ()  [unwired: 9 in, 2 out]
              n226 = Round To Nearest(number=w306) -> (nearest integer value=w305:dbl)
              n227 = local write "Distance From Target"(w305) -> ()
            }
          }
        }
      }
    }
  }
  n228 = Not(x=w50) -> (.not. x?=w72:bool)
  n229 = Not(x=w51) -> (.not. x?=w63:bool)
  n230 = Divide(x=w53, y="Maximum Encoder speed") -> (x/y=w43:dbl)
  n231 = Divide(x=w54, y="Maximum Encoder speed") -> (x/y=w42:dbl)
  n232 = call <vilib>:"SD Write Number.vi"("Numeric"=w9, "Name"="Distance From Target") -> ()  [unwired: 8 in, 2 out]
  n233 = call <vilib>:"SD Write String.vi"("Table Prefix"=w7, "Name"="Current Status") -> ()  [unwired: 8 in, 2 out]
  n234 = Add(x=w43, y=w42) -> (x+y=w41:dbl)
  n235 = local read "Shooter Speed"() -> (w38:dbl)
  n236 = call-poly <vilib>:"PID.vi"("reinitialize? (F)"=w72, "output range"=cluster{"output high":dbl, "output low":dbl} {"output high"=1.0, "output low"=-1.0}, "PID gains"="PID gains", "process variable"=w42, "setpoint"=w49) -> ("output"=w71:dbl)  [unwired: 5 in, 1 out]
  n237 = call-poly <vilib>:"PID.vi"("reinitialize? (F)"=w63, "output range"=cluster{"output high":dbl, "output low":dbl} {"output high"=1.0, "output low"=-1.0}, "PID gains"="PID gains", "process variable"=w43, "setpoint"=w48) -> ("output"=w62:dbl)  [unwired: 5 in, 1 out]
  n238 = Divide(x=w41, y=2.0) -> (x/y=w37:dbl)
  n239 = call <vilib>:"SD Write Number.vi"("Numeric"=w37, "Name"="Real Speed") -> ()  [unwired: 8 in, 2 out]
  n240 = call <vilib>:"SD Write Number.vi"("Numeric"=w38, "Name"="Speed Target") -> ()  [unwired: 8 in, 2 out]
  n241 = Subtract(x=w37, y=w38) -> (x-y=w36:dbl)
  n242 = call <vilib>:"WPI_MotorControlRefNum Registry Get.vi"("refnum name"="Shooter 1") -> ("MotorControlDevRef"=w65:T12)  [unwired: 9 in, 1 out]
  n243 = call <vilib>:"WPI_MotorControlRefNum Registry Get.vi"("refnum name"="Shooter 2") -> ("MotorControlDevRef"=w56:T12)  [unwired: 9 in, 1 out]
  n244 = Select(t=w71, s=w50, f=0.0) -> (s? t:f=w67:dbl)
  n245 = Select(t=w62, s=w51, f=0.0) -> (s? t:f=w58:dbl)
  n246 = Absolute Value(x=w36) -> (abs(x)=w35:dbl)
  n247 = call <vilib>:"WPI_MotorControlSetOutput.vi"("Output"=w67, "MotorControlDevRef"=w65) -> ()  [unwired: 7 in, 3 out]
  n248 = call <vilib>:"WPI_MotorControlSetOutput.vi"("Output"=w58, "MotorControlDevRef"=w56) -> ()  [unwired: 7 in, 3 out]
  n249 = Less?(x=w35, y="Threshold for shooter") -> (x < y?=w33:bool)
  n250 = call <vilib>:"SD Write Boolean.vi"("Boolean"=w33, "Name"="Ready to Shoot?") -> ()  [unwired: 8 in, 2 out]
  n251 = local write "Ready To Fire"(w33) -> ()
  n252 = case shown="True" "Boolean" {
    frame False {
    }
    frame True {
      n253 = call <vilib>:"WPI_EncoderRefNum Registry Get.vi"("refnum name"="Encoder On Right") -> ("error out"=w320:errorcluster, "EncoderDevRef"=w321:T4)  [unwired: 9 in]
      n254 = call <vilib>:"WPI_EncoderRefNum Registry Get.vi"("refnum name"="Encoder On Left") -> ("error out"=w318:errorcluster, "EncoderDevRef"=w319:T4)  [unwired: 9 in]
      n255 = call <vilib>:"WPI_EncoderReset.vi"("error in (no error)"=w320, "EncoderDevRef"=w321) -> ()  [unwired: 8 in, 2 out]
      n256 = call <vilib>:"WPI_EncoderReset.vi"("error in (no error)"=w318, "EncoderDevRef"=w319) -> ()  [unwired: 8 in, 2 out]
    }
  }
